vi "lab session 5.vi"() -> ()   [LabVIEW 2020]
panel:
  in  "stop":bool
  out "msg indicator":bool
  out "iterations":dbl
  out "value generated":dbl
  out "Numeric":dbl
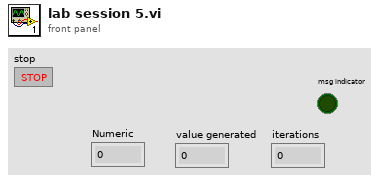
[diagram p1: front panel]
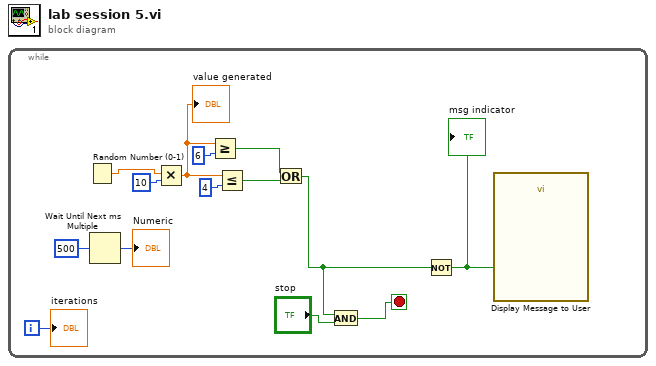
[diagram p0: block diagram]
diagram:
  n1 = while {
    i -> [w11]
    stop <- w3 stop-if-true
    n2 = Random Number (0-1)() -> (number: 0 to 1=w5:dbl)
    n3 = Wait Until Next ms Multiple(millisecond multiple=u32 500) -> (millisecond timer value=→"Numeric":u32)
    n4 = Multiply(x=w5, y=u64 10 ("lower bound (0)")) -> (x*y=w8:dbl)
    "value generated" <- w8
    n5 = Greater Or Equal?(x=w8, y=u64 6 ("lower bound (0)")) -> (x >= y?=w6:bool)
    n6 = Less Or Equal?(x=w8, y=u64 4 ("lower bound (0)")) -> (x <= y?=w7:bool)
    n7 = Or(x=w6, y=w7) -> (x .or. y?=w2:bool)
    n8 = And(x=w2, y="stop") -> (x .and. y?=w3:bool)
    n9 = Not(x=w2) -> (.not. x?=w1:bool)
    "msg indicator" <- w1
    n10 = call "Display Message to User"("Enable"=w1) -> ()  [unwired: 9 in, 2 out]
    "iterations" <- w11
  }
